vi "lo creat.vi"(8 "error in (no error)":errorcluster, 10 "mode":i32) -> (0 "error out":errorcluster, 2 "lo_creat":u32)   [LabVIEW 2019, in "libpqlv64.lvlib"]
uses:
  libpqlv64.lvlib
  libpq.dll
panel:
  in  "conn":u32
  out "conn_out":u32
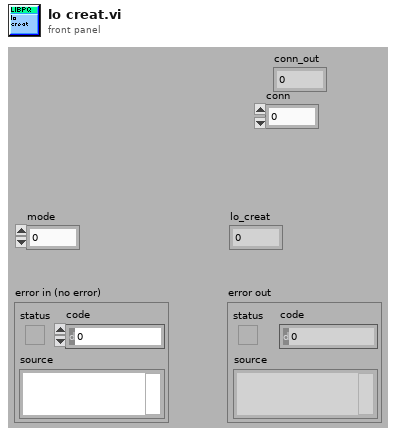
[diagram p1: front panel]
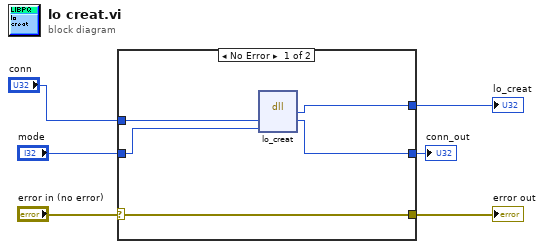
[diagram p0: block diagram]
diagram:
  n1 = case shown="No Error" "error in (no error)" {
    selector: "error in (no error)" -> [w11 w13]
    tunnel: [w11 w13] -> w5
    tunnel: [w10 _] -> w4
    tunnel: [w8 w12] -> w2
    tunnel: "mode" -> [w9 _]
    tunnel: "conn" -> [w7 w12]
    frame No Error {
      n2 = dll-call lib="libpq.*" fn="lo_creat"("conn"=w7, "mode"=w9) -> ("lo_creat"=w10:u32, "conn"=w8:u32)  [unwired: 4 in, 2 out]
    }
    frame Error {
    }
  }
  "lo_creat" <- w4
  "error out" <- w5
  "conn_out" <- w2
